vi "Read Meta Data.vi"(7 "Linked List ID":string, 8 "error in (no error)":errorcluster, 11 "Linked List Ref":refnum<data-value>) -> (0 "error out":errorcluster, 1 "Found?":bool, 2 "Meta Data":string, 3 "Linked List Ref out":refnum<data-value>)   [LabVIEW 2017, in "Linked Lists.lvlib" / "Linked List Ref.lvclass"]
uses:
  <vilib>/gpm_packages/@cs/linked-list/Source/Linked List/Linked List Ref/Linked List Ref.lvclass
  <vilib>/gpm_packages/@cs/linked-list/Source/Linked List/ILinkedList/ILinked List.lvclass
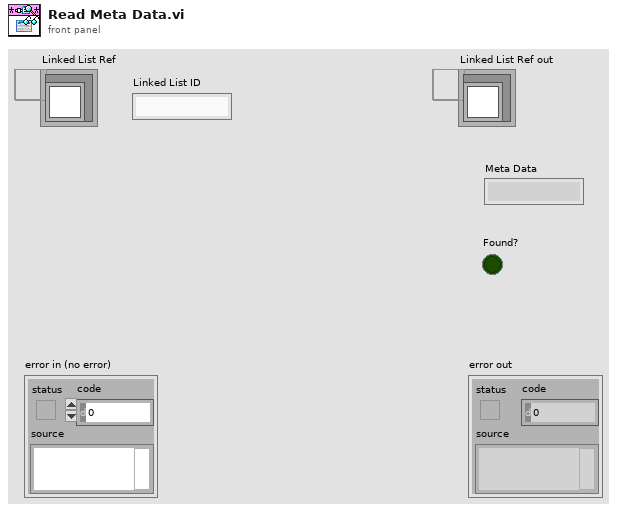
[diagram p1: front panel]
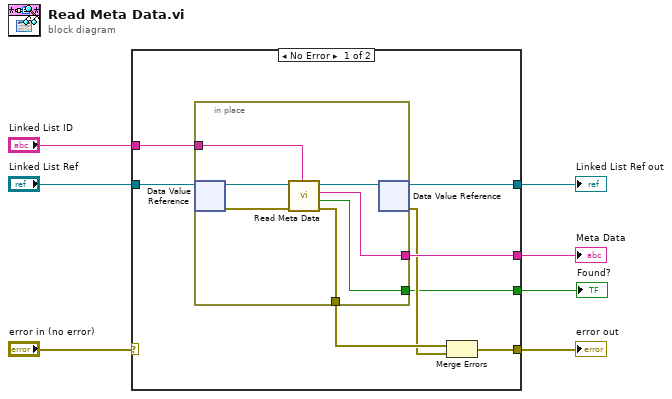
[diagram p0: block diagram]
diagram:
  n1 = case shown="No Error" "error in (no error)" {
    selector: "error in (no error)" -> [_ w24]
    tunnel: "Linked List Ref" -> [w15 w23]
    tunnel: "Linked List ID" -> [w14 _]
    tunnel: [w12 w24] -> w4
    tunnel: [w13 w23] -> w3
    tunnel: [w10 _] -> w2
    tunnel: [w8 _] -> w1
    frame No Error {
      n2 = in-place {
        in-place-border: w14 -> [w21]
        in-place-border: [w17] -> w11
        in-place-border: [w18] -> w10
        in-place-border: [w16] -> w8
        n3 = in-place-dvr #1(w15) -> (w22:refnum<class "ILinked List.lvclass">, w20:errorcluster)
        n4 = call-dynamic "Read Meta Data.vi"("Linked List ID"=w21, "error in (no error)"=w20, "ILinked List in"=w22) -> ("error out"=w17:errorcluster, "Found?"=w16:bool, "Meta Data"=w18:string, "ILinked List out"=w19:refnum<class "ILinked List.lvclass">)  [unwired: 5 in]
        n5 = in-place-dvr #1(w19) -> (w13:refnum<data-value>, w9:errorcluster)
      }
      n6 = Merge Errors(w11, w9) -> (w12:errorcluster)
    }
    frame Error {
    }
  }
  "error out" <- w4
  "Linked List Ref out" <- w3
  "Meta Data" <- w2
  "Found?" <- w1
